vi "Store Operators (SubVI).vi"(7 "Operator Command":T2=enum."Clear", 8 "error in":errorcluster, 11 "Operator":string) -> (0 "error out":errorcluster, 3 "Operator Array":T1[](array[typedef]))   [LabVIEW 2012]
doc: "FGV for operators (defined by the Operator String Control.ctl)\n\nBuild - Builds an operator into the operator array\nGET - Returns the operator array stored in the shift register\nClear - Stores an empty array"
uses:
  Controls/Operator Types.ctl
  Controls/Operator String Control.ctl
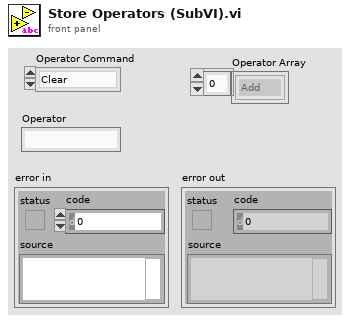
[diagram p1: front panel]
types:
  T1 = typedef "Operator Types.ctl" = enum16{"Add", "Subtract", "Multiply", "Divide"}
  T2 = typedef "Operator String Control.ctl" = enum16{"GET", "Build", "Clear"}
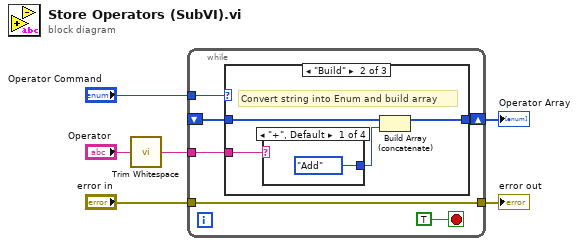
[diagram p0: block diagram]
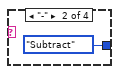
[diagram p3: hidden frame]
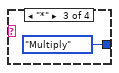
[diagram p4: hidden frame]
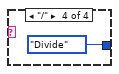
[diagram p5: hidden frame]
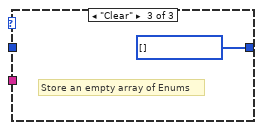
[diagram p6: hidden frame]
diagram:
  n1 = call <vilib>:"Trim Whitespace.vi"("string"="Operator") -> ("trimmed string"=w3:string)  [unwired: 1 in]
  n2 = while {
    tunnel: "error in" -> [w11]
    tunnel: [w11] -> w4
    tunnel: "Operator Command" -> [w10]
    tunnel: w3 -> [w7]
    shift-right: [w9] -> w2
    shift-left: _ -> [w8]
    stop <- TRUE stop-if-true
    n3 = case shown="\"Build\"" w10 {
      tunnel: [w13 w15 w22] -> w9
      tunnel: w8 -> [w13 w14 _]
      tunnel: w7 -> [_ w17 _]
      frame "GET" {
        # "Return the operator array"
      }
      frame "Build" {
        # "Convert string into Enum and build array"
        n4 = case shown="\"+\", Default" w17 {
          tunnel: [Operator_Types."Add" ("Enum") Operator_Types."Subtract" ("Enum") Operator_Types."Multiply" ("Enum") Operator_Types."Divide" ("Enum")] -> w16
          frame "+", Default {
          }
          frame "-" {
          }
          frame "*" {
          }
          frame "/" {
          }
        }
        n5 = Build Array (concatenate)(w14, w16) -> (w15:T1[])
      }
      frame "Clear" {
        w22 = T1[] [] items=["Add", "Subtract", "Multiply", "Divide"]
        # "Store an empty array of Enums"
      }
    }
  }
  "error out" <- w4
  "Operator Array" <- w2
